vi "exercice2-2.vi"() -> ()   [LabVIEW 2013]
panel:
  out "Booléen 6":bool
  out "Booléen 5":bool
  out "Booléen 4":bool
  in  "Booléen 3":bool
  in  "Booléen 2":bool
  in  "Booléen":bool
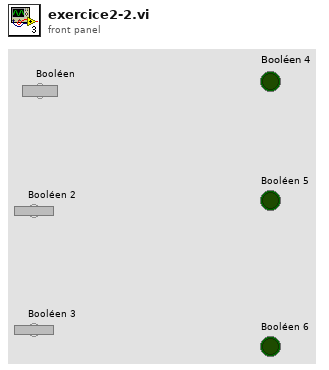
[diagram p1: front panel]
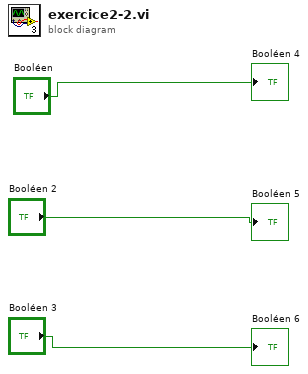
[diagram p0: block diagram]
diagram:
  "Booléen 4" <- "Booléen"
  "Booléen 5" <- "Booléen 2"
  "Booléen 6" <- "Booléen 3"
